vi "SubVI_Close_TCP_Connection.vi"(8 "error in (no error)":errorcluster, 11 "TCP Network Connection in":refnum<k5>) -> (0 "error out":errorcluster, 3 "Case to Switch to following Close":i32)   [LabVIEW 2020]
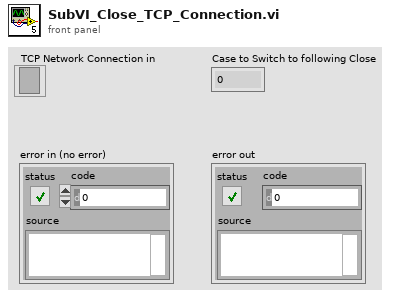
[diagram p1: front panel]
types:
  T1 = enum16{"Standard", "Buffered", "CRLF", "Immediate"}
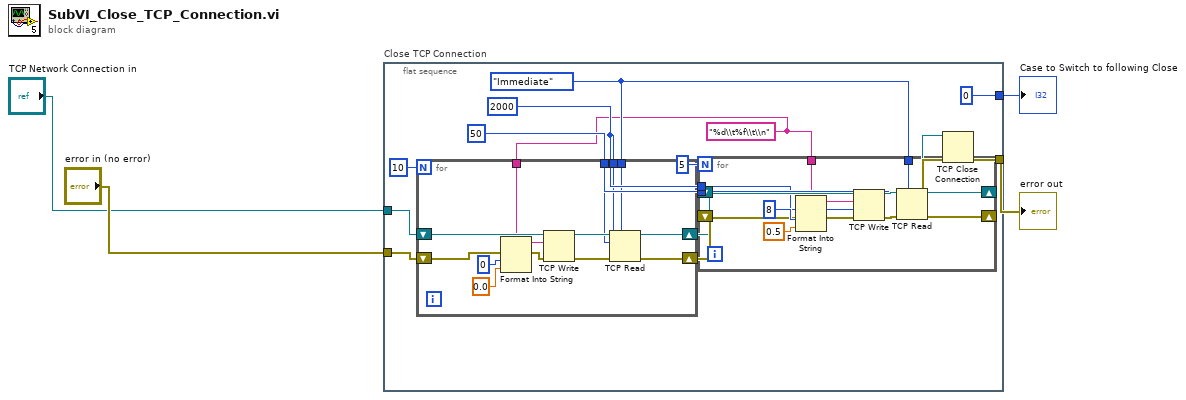
[diagram p0: block diagram]
diagram:
  n1 = flat-sequence "Close TCP Connection" {
    tunnel: "error in (no error)" -> [w14]
    tunnel: "TCP Network Connection in" -> [w13]
    tunnel: [w16] -> w3
    tunnel: [0 ("Tab Select")] -> w4
    frame #0 {
      w5 = "%d\\t%f\\t\\n" ("format string")
      w8 = 2000 ("timeout ms (25000)")
      w9 = T1."Immediate" ("mode (standard)")
      w12 = 50 ("bytes to read")
      n2 = for {
        N: 10 -> [_]
        tunnel: w12 -> [w37]
        tunnel: w9 -> [w34]
        tunnel: w8 -> [w33]
        shift-right: [w36] -> w11
        shift-left: w14 -> [w43]
        shift-right: [w35] -> w10
        shift-left: w13 -> [w41]
        tunnel: w5 -> [w32]
        n3 = Format Into String(format string=w32, error in=w43, 0 ("input 1"), 0.0) -> (resulting string=w42:string, error out=w40:errorcluster)  [unwired: 1 in]
        n4 = TCP Write(connection ID=w41, data in=w42, error in (no error)=w40) -> (connection ID out=w38:refnum<k5>, error out=w39:errorcluster)  [unwired: 1 in, 1 out]
        n5 = TCP Read(connection ID=w38, bytes to read=w37, error in (no error)=w39, 7:w34, 9:w33) -> (connection ID out=w35:refnum<k5>, error out=w36:errorcluster)  [unwired: 1 out]
      }
      n6 = for {
        N: 5 -> [_]
        tunnel: w12 -> [w24]
        tunnel: w9 -> [w21]
        tunnel: w8 -> [w20]
        shift-right: [w26] -> w18
        shift-left: w11 -> [w23]
        shift-right: [w25] -> w17
        shift-left: w10 -> [w22]
        tunnel: w5 -> [w19]
        n7 = Format Into String(format string=w19, 8 ("input 1"), 0.5) -> (resulting string=w29:string)  [unwired: 2 in, 1 out]
        n8 = TCP Write(connection ID=w22, data in=w29, error in (no error)=w23, 9:w20) -> (connection ID out=w27:refnum<k5>, error out=w28:errorcluster)  [unwired: 1 out]
        n9 = TCP Read(connection ID=w27, bytes to read=w24, error in (no error)=w28, 7:w21) -> (connection ID out=w25:refnum<k5>, error out=w26:errorcluster)  [unwired: 1 in, 1 out]
      }
      n10 = TCP Close Connection(connection ID=w17, error in (no error)=w18) -> (error out=w16:errorcluster)  [unwired: 1 in, 1 out]
    }
  }
  "Case to Switch to following Close" <- w4
  "error out" <- w3
